vi "API Motor Stop.vi"(10 "motorNum":i32) -> (3 "motorstop return value":bool)   [LabVIEW 2011, in "API DYM.lvlib"]
uses:
  API DYM.lvlib
  DyMechnicalPlatform.dll
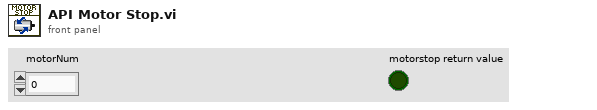
[diagram p1: front panel]
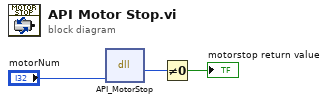
[diagram p0: block diagram]
diagram:
  n1 = dll-call lib="D:/Documents/GitHub/DYSYS/DYSYS/API/DyMechnicalPlatform.dll" fn="API_MotorStop"("motorNum"="motorNum") -> ("返回类型"=w2:i32)  [unwired: 4 in, 2 out]
  n2 = Not Equal To 0?(x=w2) -> (x != 0?=→"motorstop return value":bool)
